vi "Dialog Condition Server.vi"() -> ()   [LabVIEW 2019, in "OPC UA Demo.lvlib"]
doc: "Demonstrates the use of the <B>OPC UA Dialog Condition </B>functionality as an OPC UA \nserver."
uses:
  OPC UA Demo.lvlib
  <vilib>/OPCUA/controls/NodeId.ctl
  <vilib>/OPCUA/controls/Data Type.ctl
  <vilib>/OPCUA/server/Add Dialog Condition.vi
  <vilib>/OPCUA/server/Write Bool.vi
  <vilib>/OPCUA/NI OPC UA Server.lvlib
panel:
  in  "stop":bool
  in  "temperature":dbl(slide) scale=0.0..100.0
  out "server endpoint URL":string
  # "Overview: Demonstrates the use of the OPC UA Dialog Condition functionality as an OPC UA \nserver.\nRequirements: \n1. LabVIEW OPC UA Toolkit\n2. Run this VI on RT targets or Windows\nInstructions:\n1. Run the VI.\n2. Run Dialog Condition Client.vi in OPC UA Demo.lvproj.\n3. When the temperature exceeds 50, the OPC UA server will trigger a dialog condition event."
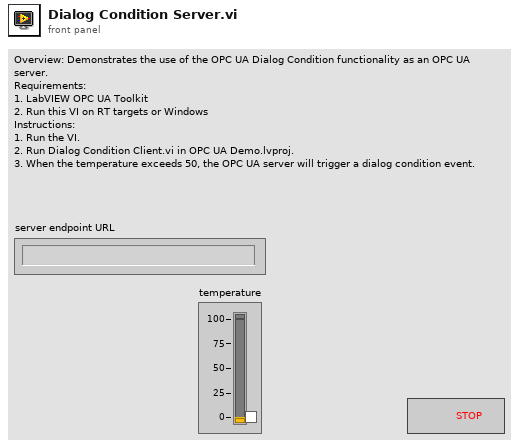
[diagram p1: front panel]
types:
  T1 = typedef "Data Type.ctl" = u16
  T2 = cluster{"name":string, "data type":T1, "access level":u16, "description":string}
  T3 = typedef "NodeId.ctl" = string
  T4 = cluster{"condition name":string, "source node ID":T3, "prompt":string, "description":string}
  T5 = typedef "OPC UA Server Refnum.ctl" = refnum<k21>
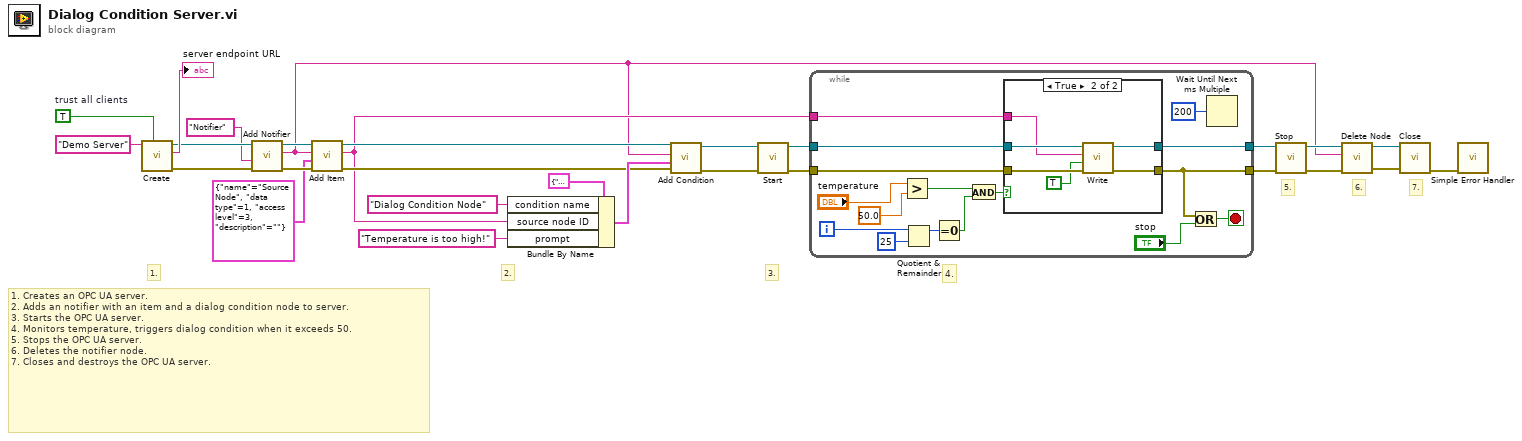
[diagram p0: block diagram]
diagram:
  w1 = TRUE  # trust all clients
  # "7."
  # "6."
  # "5."
  # "4."
  # "3."
  # "2."
  # "1."
  # "1. Creates an OPC UA server.\n2. Adds an notifier with an item and a dialog condition node to server.\n3. Starts the OPC UA server.\n4. Monitors temperature, triggers dialog condition when it exceeds 50. \n5. Stops the OPC UA server.\n6. Deletes the notifier node.\n7. Closes and destroys the OPC UA server."
  n1 = call <vilib>:"Create.vi"("trust all clients (F)"=w1, "OPC UA server name"="Demo Server") -> ("error out"=w25:errorcluster, "server endpoint URL"=→"server endpoint URL":string, "OPC UA server refnum out"=w26:T5)  [unwired: 7 in]
  n2 = call <vilib>:"Add Notifier.vi"("error in (no error)"=w25, "notifier name"="Notifier" ("folder name"), "OPC UA server refnum in"=w26) -> ("error out"=w23:errorcluster, "notifier node ID"=w2:T3, "OPC UA server refnum out"=w24:T5)  [unwired: 4 in, 1 out]
  n3 = call <vilib>:"Add Item.vi"("error in (no error)"=w23, "item"=T2 {"name"="Source Node", "data type"=1, "access level"=3, "description"=""}, "parent folder node ID"=w2, "OPC UA server refnum in"=w24) -> ("error out"=w15:errorcluster, "item node ID"=w12:T3, "OPC UA server refnum out"=w16:T5)  [unwired: 3 in, 1 out]
  n4 = Bundle By Name(cluster=T4 {"condition name"="", "source node ID"="", "prompt"="", "description"=""} ("property"), "condition name"="Dialog Condition Node", "source node ID"=w12, "prompt"="Temperature is too high!") -> (w19:T4)
  n5 = call-poly <vilib>:"Add Condition.vi"("error in (no error)"=w15, "property"=w19, "notifier node ID"=w2, "OPC UA server refnum in"=w16) -> ("error out"=w17:errorcluster, "OPC UA server refnum out"=w18:T5)  [unwired: 4 in, 2 out]
  n6 = call <vilib>:"Start.vi"("error in (no error)"=w17, "OPC UA server refnum in"=w18) -> ("error out"=w13:errorcluster, "OPC UA server refnum out"=w14:T5)  [unwired: 7 in, 1 out]
  n7 = while {
    tunnel: w14 -> [w44]
    tunnel: w13 -> [w43]
    tunnel: w12 -> [w41]
    tunnel: [w42] -> w11
    tunnel: [w38] -> w10
    i -> [w34]
    stop <- w36 stop-if-true
    n8 = Greater?(x="temperature", y=50.0) -> (0:w32:bool)
    n9 = Quotient & Remainder(x=w34, y=25) -> (x-y*floor(x/y)=w30:i32)  [unwired: 1 out]
    n10 = Equal To 0?(x=w30) -> (x = 0?=w29:bool)
    n11 = And(x=w32, y=w29) -> (x .and. y?=w31:bool)
    n12 = case shown="True" w31 {
      tunnel: w44 -> [w46 w52]
      tunnel: w43 -> [w45 w51]
      tunnel: [w46 w50] -> w42
      tunnel: [w45 w49] -> w38
      tunnel: w41 -> [_ w48]
      frame False {
      }
      frame True {
        n13 = call-poly <vilib>:"Write.vi"("error in (no error)"=w51, "value"=TRUE, "node ID"=w48, "OPC UA server refnum in"=w52) -> ("error out"=w49:errorcluster, "OPC UA server refnum out"=w50:T5)  [unwired: 5 in, 1 out]
      }
    }
    n14 = Or(x=w38, y="stop") -> (x .or. y?=w36:bool)
    n15 = Wait Until Next ms Multiple(millisecond multiple=u32 200) -> ()  [unwired: 1 out]
  }
  n16 = call <vilib>:"Stop.vi"("error in (no error)"=w10, "OPC UA server refnum in"=w11) -> ("error out"=w7:errorcluster, "OPC UA server refnum out"=w8:T5)  [unwired: 8 in]
  n17 = call <vilib>:"Delete Node.vi"("error in (no error)"=w7, "node ID"=w2, "OPC UA server refnum in"=w8) -> ("error out"=w5:errorcluster, "OPC UA server refnum out"=w6:T5)  [unwired: 7 in]
  n18 = call <vilib>:"Close.vi"("error in (no error)"=w5, "OPC UA server refnum in"=w6) -> ("error out"=w9:errorcluster)  [unwired: 9 in]
  n19 = call <vilib>:"Simple Error Handler.vi"("error in (no error)"=w9) -> ()  [unwired: 4 in, 5 out]
